vi "GetCommandsFromFile.vi"(8 "error in":errorcluster, 9 "CommandQueue":refnum<queue>, 10 "DeviceControlQueue":refnum<queue>, 11 "Path":path) -> (0 "error out":errorcluster)   [LabVIEW 2017]
uses:
  CommandCluster.ctl
  Utilities/WordManipulationLibrary.lvlib
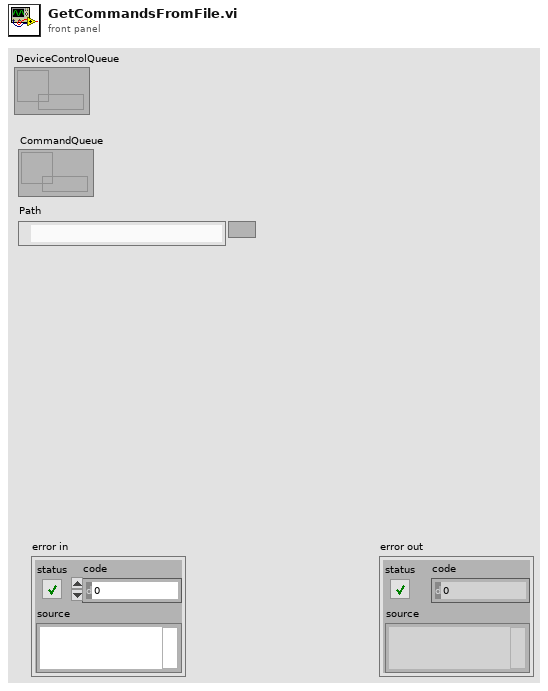
[diagram p1: front panel]
types:
  T1 = enum16{"Shutdown", "Switch On", "Disable Voltage", "Quick Stop", "Disable Op", "Enable Op", "Fault Reset", "Error"}[]
  T2 = enum16{"Reserved", "Profile Position Mode", "Velocity Mode", "Profile Velocity Mode", "Profile Torque Mode", "Reserved 2", "Reference Mode", "Interpolated Position Mode", "Skip"}
  T3 = typedef "CommandCluster.ctl" = cluster{"Modes":enum16{"Reserved", "Profile Position Mode", "Velocity Mode", "Profile Velocity Mode", "Profile Torque Mode", "Reserved 2", "Reference Mode", "Interpolated Position Mode", "Skip"}, "Parameters_PositionProfile":dbl[]}
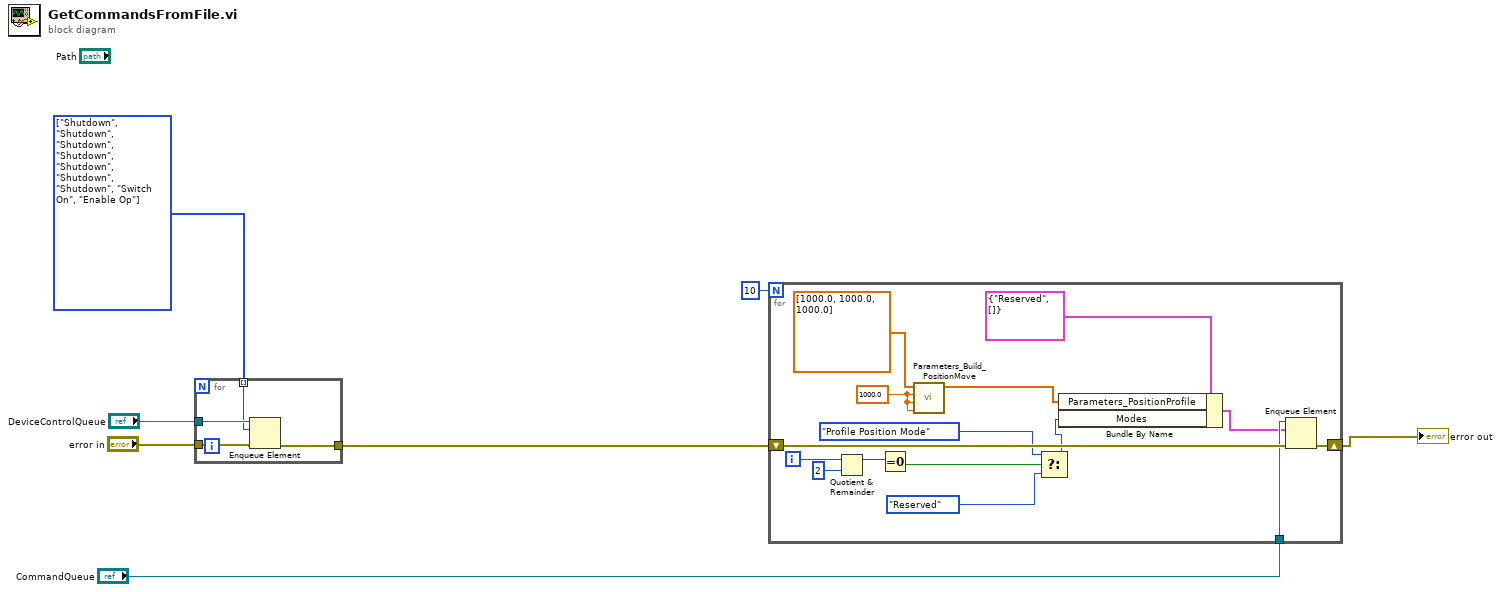
[diagram p0: block diagram]
diagram:
  w5 = T1 [enum."Shutdown", enum."Shutdown", enum."Shutdown", enum."Shutdown", enum."Shutdown", enum."Shutdown", enum."Shutdown", enum."Switch On", enum."Enable Op"] items=["Shutdown", "Switch On", "Disable Voltage", "Quick Stop", "Disable Op", "Enable Op", "Fault Reset", "Error"] ("Device Control")
  n1 = for {
    tunnel: "error in" -> [w11]
    tunnel: "DeviceControlQueue" -> [w10]
    tunnel: w5 -> [w9] mode=indexing
    tunnel: [w8] -> w4
    n2 = Enqueue Element(queue=w10, element=w9, error in (no error)=w11) -> (error out=w8:errorcluster)  [unwired: 1 in, 2 out]
  }
  n3 = for {
    N: 10 -> [_]
    shift-right: [w24] -> w1
    shift-left: w4 -> [w25]
    tunnel: "CommandQueue" -> [w23]
    i -> [w18]
    w20 = 1000.0 ("Velocity")
    n4 = Quotient & Remainder(x=w18, y=2) -> (x-y*floor(x/y)=w16:i32)  [unwired: 1 out]
    n5 = Equal To 0?(x=w16) -> (x = 0?=w12:bool)
    n6 = call "Parameters_Build_PositionMove.vi"("Acceleration Jerk"=w20, "Acceleration"=w20, "Velocity"=w20, "Positions"=dbl[] [1000.0, 1000.0, 1000.0]) -> ("Parameters"=w21:dbl[])  [unwired: 7 in]
    n7 = Select(t=T2."Profile Position Mode" ("Modes"), s=w12, f=T2."Reserved" ("Modes")) -> (s? t:f=w14:T2)
    n8 = Bundle By Name(cluster=T3 {"Modes"=enum."Reserved", "Parameters_PositionProfile"=[]} ("element"), "Parameters_PositionProfile"=w21, "Modes"=w14) -> (w19:T3)
    n9 = Enqueue Element(queue=w23, element=w19, error in (no error)=w25) -> (error out=w24:errorcluster)  [unwired: 1 in, 2 out]
  }
  "error out" <- w1
